vi "LaneExtractorHenesUseNetwork.vi"() -> ()   [LabVIEW 2024]
uses:
  <vilib>/userDefined/High Color/IMAQdx.ctl
  System.Windows.Forms
  <vilib>/Instr/_visa.llb/VISA Set IO Buffer Mask.ctl
  <vilib>/Instr/_visa.llb/VISA Flush IO Buffer Mask.ctl
  7dfa5429-d58f-460b-bb70-c7f4b3dcb04f.vi
  <vilib>/Instr/_visa.llb/VISA Configure Serial Port (Instr).vi
  <vilib>/Python/Open Venv Python Session.vi
  <vilib>/vision/driver/NI_Vision_Acquisition_Software.lvlib
panel:
  out "error out 2":errorcluster
  out "error out":errorcluster
  out "session out":refnum<k35>
  in  "ctelim":dbl=0.3 format="%#_13g"
  in  "GoBack":bool
  in  "Threshold":i32=1900
  in  "Spacing":i32=100
  in  "eps":i32=100
  in  "min_samples":i32=2
  in  "Ratio_Threshold":i32=4
  out "X_arrays":dbl[](array[numeric])=[-1100.0, -1100.0, -1120.0, -1120.0, -1140.0, -1140.0, -1140.0, -1160.0, -1160.0, -1160.0, -1180.0, -1180.0, -1180.0, -1200.0, -1200.0, -1200.0, -1220.0, -1220.0, -1220.0, -1220.0, -1240.0, -1260.0, -1260.0, -1260.0, -1280.0, -1280.0, -1280.0, -1300.0, -1300.0, -1300.0, -1320.0, -1320.0, -1320.0, -1340.0, -1340.0, -1340.0, -1360.0, -1360.0, -1360.0, -1380.0, -1380.0, -1380.0, -1400.0, -1400.0, -1400.0, -1420.0, -1420.0, -1440.0, -1440.0, -1460.0, -1460.0, -1460.0, -1480.0, -1480.0, -1480.0, -1480.0, -1500.0, -1500.0, -1500.0, -1520.0, -1520.0, -1520.0, -1540.0, -1540.0, -1540.0, -1560.0, -1560.0, -1560.0, -1580.0, -1580.0, -1600.0, -1600.0, -1620.0, -1620.0, -1620.0, -1640.0, -1640.0, -1640.0, -1660.0, -1660.0, -1680.0, -1680.0, -1680.0, -1700.0, -1700.0, -1700.0, -1720.0, -1720.0, -1740.0, -1740.0, -1760.0, -1760.0, -1780.0, -1780.0, -1780.0, -1800.0, -1820.0, -1820.0, -1820.0, -1840.0, -1840.0, -1860.0, -1860.0, -1880.0, -1880.0, -1900.0, -1900.0, -1920.0, -1940.0, -1960.0, -1960.0, -1980.0, -2000.0, -2000.0, -2040.0, -2060.0, -2060.0, -2080.0, -2120.0, -2120.0, -2140.0, -2140.0, -2160.0, -2180.0, -2200.0, -2220.0, -2220.0, -2260.0, -2280.0, -2300.0, -2320.0, -2340.0, -2360.0, -2380.0, -2400.0, -2420.0, -2460.0, -2500.0, -2520.0, -2540.0, -2580.0, -2980.0, -2980.0, -2960.0, -2940.0, -2960.0, 1180.0, 1200.0, 1220.0, 1220.0, 1240.0, 1260.0, 1260.0, 1280.0, 1380.0, 1380.0, 1380.0, 1400.0, 1400.0, 1420.0, 1420.0, 1440.0, 1460.0, 3460.0, 3460.0, 3460.0, 3460.0, 3460.0, 3480.0, 3480.0, 3500.0, -1657.163120567376, -2964.0, 1232.5, 1408.888888888889, 3470.0, 1252.0987654320988, 1271.6975308641975, 1291.2962962962963, 1310.8950617283951, 1330.4938271604938, 1350.0925925925926, 1369.6913580246915, 1389.29012345679]
  out "Y_arrays":dbl[](array[numeric])=[40.0, 60.0, 60.0, 80.0, 80.0, 100.0, 120.0, 120.0, 140.0, 160.0, 180.0, 200.0, 220.0, 220.0, 240.0, 260.0, 260.0, 280.0, 300.0, 320.0, 340.0, 360.0, 380.0, 400.0, 420.0, 440.0, 460.0, 460.0, 480.0, 500.0, 520.0, 540.0, 560.0, 560.0, 580.0, 600.0, 620.0, 640.0, 660.0, 660.0, 680.0, 700.0, 700.0, 720.0, 740.0, 760.0, 780.0, 800.0, 820.0, 840.0, 860.0, 880.0, 880.0, 900.0, 920.0, 940.0, 940.0, 960.0, 980.0, 980.0, 1000.0, 1020.0, 1020.0, 1040.0, 1060.0, 1080.0, 1100.0, 1120.0, 1140.0, 1160.0, 1180.0, 1200.0, 1220.0, 1240.0, 1260.0, 1260.0, 1280.0, 1300.0, 1320.0, 1340.0, 1360.0, 1380.0, 1400.0, 1420.0, 1440.0, 1460.0, 1480.0, 1500.0, 1520.0, 1540.0, 1560.0, 1580.0, 1600.0, 1620.0, 1640.0, 1660.0, 1700.0, 1720.0, 1740.0, 1760.0, 1780.0, 1800.0, 1820.0, 1860.0, 1880.0, 1900.0, 1940.0, 1960.0, 2000.0, 2040.0, 2080.0, 2120.0, 2140.0, 2160.0, 2240.0, 2260.0, 2300.0, 2340.0, 2400.0, 2420.0, 2460.0, 2480.0, 2520.0, 2560.0, 2600.0, 2660.0, 2700.0, 2740.0, 2800.0, 2840.0, 2880.0, 2940.0, 3000.0, 3060.0, 3100.0, 3160.0, 3240.0, 3300.0, 3360.0, 3420.0, 3500.0, 4340.0, 4360.0, 4380.0, 4380.0, 4460.0, 2560.0, 2580.0, 2560.0, 2540.0, 2540.0, 2540.0, 2520.0, 2520.0, 1720.0, 1700.0, 1680.0, 1680.0, 1660.0, 1660.0, 1640.0, 1660.0, 1660.0, 1800.0, 1780.0, 1760.0, 1740.0, 1720.0, 1720.0, 1700.0, 1700.0, 1330.354609929078, 4384.0, 2545.0, 1673.3333333333333, 1740.0, 2448.1481481481483, 2351.296296296296, 2254.4444444444443, 2157.5925925925926, 2060.740740740741, 1963.888888888889, 1867.037037037037, 1770.1851851851852]
  out "Clustered":T1={"appended array"=[-1100.0, -1100.0, -1120.0, -1120.0, -1140.0, -1140.0, -1140.0, -1160.0, -1160.0, -1160.0, -1180.0, -1180.0, -1180.0, -1200.0, -1200.0, -1200.0, -1220.0, -1220.0, -1220.0, -1220.0, -1240.0, -1260.0, -1260.0, -1260.0, -1280.0, -1280.0, -1280.0, -1300.0, -1300.0, -1300.0, -1320.0, -1320.0, -1320.0, -1340.0, -1340.0, -1340.0, -1360.0, -1360.0, -1360.0, -1380.0, -1380.0, -1380.0, -1400.0, -1400.0, -1400.0, -1420.0, -1420.0, -1440.0, -1440.0, -1460.0, -1460.0, -1460.0, -1480.0, -1480.0, -1480.0, -1480.0, -1500.0, -1500.0, -1500.0, -1520.0, -1520.0, -1520.0, -1540.0, -1540.0, -1540.0, -1560.0, -1560.0, -1560.0, -1580.0, -1580.0, -1600.0, -1600.0, -1620.0, -1620.0, -1620.0, -1640.0, -1640.0, -1640.0, -1660.0, -1660.0, -1680.0, -1680.0, -1680.0, -1700.0, -1700.0, -1700.0, -1720.0, -1720.0, -1740.0, -1740.0, -1760.0, -1760.0, -1780.0, -1780.0, -1780.0, -1800.0, -1820.0, -1820.0, -1820.0, -1840.0, -1840.0, -1860.0, -1860.0, -1880.0, -1880.0, -1900.0, -1900.0, -1920.0, -1940.0, -1960.0, -1960.0, -1980.0, -2000.0, -2000.0, -2040.0, -2060.0, -2060.0, -2080.0, -2120.0, -2120.0, -2140.0, -2140.0, -2160.0, -2180.0, -2200.0, -2220.0, -2220.0, -2260.0, -2280.0, -2300.0, -2320.0, -2340.0, -2360.0, -2380.0, -2400.0, -2420.0, -2460.0, -2500.0, -2520.0, -2540.0, -2580.0, -2980.0, -2980.0, -2960.0, -2940.0, -2960.0, 1180.0, 1200.0, 1220.0, 1220.0, 1240.0, 1260.0, 1260.0, 1280.0, 1380.0, 1380.0, 1380.0, 1400.0, 1400.0, 1420.0, 1420.0, 1440.0, 1460.0, 3460.0, 3460.0, 3460.0, 3460.0, 3460.0, 3480.0, 3480.0, 3500.0, -1657.163120567376, -2964.0, 1232.5, 1408.888888888889, 3470.0, 1252.0987654320988, 1271.6975308641975, 1291.2962962962963, 1310.8950617283951, 1330.4938271604938, 1350.0925925925926, 1369.6913580246915, 1389.29012345679], "appended array"=[40.0, 60.0, 60.0, 80.0, 80.0, 100.0, 120.0, 120.0, 140.0, 160.0, 180.0, 200.0, 220.0, 220.0, 240.0, 260.0, 260.0, 280.0, 300.0, 320.0, 340.0, 360.0, 380.0, 400.0, 420.0, 440.0, 460.0, 460.0, 480.0, 500.0, 520.0, 540.0, 560.0, 560.0, 580.0, 600.0, 620.0, 640.0, 660.0, 660.0, 680.0, 700.0, 700.0, 720.0, 740.0, 760.0, 780.0, 800.0, 820.0, 840.0, 860.0, 880.0, 880.0, 900.0, 920.0, 940.0, 940.0, 960.0, 980.0, 980.0, 1000.0, 1020.0, 1020.0, 1040.0, 1060.0, 1080.0, 1100.0, 1120.0, 1140.0, 1160.0, 1180.0, 1200.0, 1220.0, 1240.0, 1260.0, 1260.0, 1280.0, 1300.0, 1320.0, 1340.0, 1360.0, 1380.0, 1400.0, 1420.0, 1440.0, 1460.0, 1480.0, 1500.0, 1520.0, 1540.0, 1560.0, 1580.0, 1600.0, 1620.0, 1640.0, 1660.0, 1700.0, 1720.0, 1740.0, 1760.0, 1780.0, 1800.0, 1820.0, 1860.0, 1880.0, 1900.0, 1940.0, 1960.0, 2000.0, 2040.0, 2080.0, 2120.0, 2140.0, 2160.0, 2240.0, 2260.0, 2300.0, 2340.0, 2400.0, 2420.0, 2460.0, 2480.0, 2520.0, 2560.0, 2600.0, 2660.0, 2700.0, 2740.0, 2800.0, 2840.0, 2880.0, 2940.0, 3000.0, 3060.0, 3100.0, 3160.0, 3240.0, 3300.0, 3360.0, 3420.0, 3500.0, 4340.0, 4360.0, 4380.0, 4380.0, 4460.0, 2560.0, 2580.0, 2560.0, 2540.0, 2540.0, 2540.0, 2520.0, 2520.0, 1720.0, 1700.0, 1680.0, 1680.0, 1660.0, 1660.0, 1640.0, 1660.0, 1660.0, 1800.0, 1780.0, 1760.0, 1740.0, 1720.0, 1720.0, 1700.0, 1700.0, 1330.354609929078, 4384.0, 2545.0, 1673.3333333333333, 1740.0, 2448.1481481481483, 2351.296296296296, 2254.4444444444443, 2157.5925925925926, 2060.740740740741, 1963.888888888889, 1867.037037037037, 1770.1851851851852]}
  out "PythonLoop":u32=100
  in  "Looking X":i32=3500
  in  "Looking Y":i32=5200
  out "LookingAt":cluster{i32[], i32[]}={[700, 700, 3500, 3500, -3500, -3500, -700, -700, 700], [800, -800, -800, 5200, 5200, -800, -800, 800, 800]}
  out "Anthena_Steer":i32
  out "TargetDerection":cluster{dbl[], dbl[]}={[4.2861222383783204e-13, 0.0], [7000.0, 0.0]}
  out "VEstop":bool
  in  "length":dbl=1300.0
  out "PointCloud":T2(graph)=[{"appended array"=[700.0, 700.0, 3500.0, 3500.0, -3500.0, -3500.0, -700.0, -700.0, 700.0], "appended array"=[800.0, -800.0, -800.0, 5200.0, 5200.0, -800.0, -800.0, 800.0, 800.0]}, {"appended array"=[-560.0], "appended array"=[0.0]}, {"appended array"=[-450.0, -450.0, -800.0, -800.0, 0.0, 0.0, -450.0], "appended array"=[100.0, -300.0, -300.0, 1200.0, 1200.0, 100.0, 100.0]}, {"appended array"=[], "appended array"=[]}, {"appended array"=[450.0, 450.0, 800.0, 800.0, 0.0, 0.0, 450.0], "appended array"=[100.0, -300.0, -300.0, 1200.0, 1200.0, 100.0, 100.0]}, {"appended array"=[-1100.0, -1100.0, -1120.0, -1120.0, -1140.0, -1140.0, -1140.0, -1160.0, -1160.0, -1160.0, -1180.0, -1180.0, -1180.0, -1200.0, -1200.0, -1200.0, -1220.0, -1220.0, -1220.0, -1220.0, -1240.0, -1260.0, -1260.0, -1260.0, -1280.0, -1280.0, -1280.0, -1280.0, -1300.0, -1300.0, -1300.0, -1320.0, -1320.0, -1320.0, -1340.0, -1340.0, -1340.0, -1360.0, -1360.0, -1360.0, -1380.0, -1380.0, -1380.0, -1400.0, -1400.0, -1400.0, -1420.0, -1420.0, -1420.0, -1440.0, -1440.0, -1440.0, -1460.0, -1460.0, -1460.0, -1480.0, -1480.0, -1480.0, -1500.0, -1500.0, -1500.0, -1500.0, -1520.0, -1520.0, -1520.0, -1540.0, -1540.0, -1540.0, -1560.0, -1560.0, -1560.0, -1580.0, -1580.0, -1580.0, -1600.0, -1600.0, -1600.0, -1620.0, -1620.0, -1620.0, -1640.0, -1640.0, -1660.0, -1660.0, -1680.0, -1680.0, -1680.0, -1700.0, -1700.0, -1720.0, -1720.0, -1720.0, -1740.0, -1740.0, -1760.0, -1760.0, -1760.0, -1780.0, -1780.0, -1800.0, -1800.0, -1820.0, -1820.0, -1840.0, -1840.0, -1860.0, -1860.0, -1880.0, -1880.0, -1900.0, -1920.0, -1920.0, -1940.0, -1960.0, -1980.0, -2000.0, -2020.0, -2040.0, -2040.0, -2060.0, -2060.0, -2100.0, -2120.0, -2120.0, -2120.0, -2140.0, -2160.0, -2180.0, -2200.0, -2220.0, -2240.0, -2260.0, -2280.0, -2300.0, -2320.0, -2360.0, -2380.0, -2400.0, -2440.0, -2460.0, -2480.0, -2520.0, -2520.0, -2540.0, -2980.0, -2960.0, -2960.0, -2940.0, 1180.0, 1200.0, 1220.0, 1220.0, 1240.0, 1260.0, 1260.0, 1280.0, 1380.0, 1380.0, 1380.0, 1400.0, 1400.0, 1420.0, 1420.0, 1440.0, 1460.0, 3460.0, 3460.0, 3460.0, 3460.0, 3480.0, 3480.0, 3500.0, -1646.388888888889, -2960.0, 1232.5, 1408.888888888889, 3471.4285714285716, 1252.0987654320988, 1271.6975308641975, 1291.2962962962963, 1310.8950617283951, 1330.4938271604938, 1350.0925925925926, 1369.6913580246915, 1389.29012345679], "appended array"=[40.0, 60.0, 60.0, 80.0, 80.0, 100.0, 120.0, 120.0, 140.0, 160.0, 180.0, 200.0, 220.0, 220.0, 240.0, 260.0, 260.0, 280.0, 300.0, 320.0, 340.0, 360.0, 380.0, 400.0, 400.0, 420.0, 440.0, 460.0, 460.0, 480.0, 500.0, 520.0, 540.0, 560.0, 560.0, 580.0, 600.0, 620.0, 640.0, 660.0, 660.0, 680.0, 700.0, 700.0, 720.0, 740.0, 740.0, 760.0, 780.0, 780.0, 800.0, 820.0, 840.0, 860.0, 880.0, 880.0, 900.0, 920.0, 920.0, 940.0, 960.0, 980.0, 980.0, 1000.0, 1020.0, 1020.0, 1040.0, 1060.0, 1080.0, 1100.0, 1120.0, 1120.0, 1140.0, 1160.0, 1160.0, 1180.0, 1200.0, 1220.0, 1240.0, 1260.0, 1280.0, 1300.0, 1320.0, 1340.0, 1360.0, 1380.0, 1400.0, 1420.0, 1440.0, 1460.0, 1480.0, 1500.0, 1520.0, 1540.0, 1560.0, 1580.0, 1600.0, 1620.0, 1640.0, 1660.0, 1680.0, 1700.0, 1720.0, 1740.0, 1780.0, 1800.0, 1820.0, 1840.0, 1860.0, 1920.0, 1940.0, 1980.0, 2020.0, 2080.0, 2120.0, 2160.0, 2180.0, 2220.0, 2240.0, 2280.0, 2320.0, 2360.0, 2400.0, 2420.0, 2460.0, 2500.0, 2540.0, 2580.0, 2620.0, 2680.0, 2720.0, 2780.0, 2820.0, 2880.0, 2920.0, 2980.0, 3020.0, 3080.0, 3160.0, 3220.0, 3280.0, 3340.0, 3380.0, 3440.0, 4340.0, 4360.0, 4380.0, 4420.0, 2560.0, 2580.0, 2560.0, 2540.0, 2540.0, 2540.0, 2520.0, 2520.0, 1720.0, 1700.0, 1680.0, 1680.0, 1660.0, 1660.0, 1640.0, 1660.0, 1660.0, 1800.0, 1780.0, 1760.0, 1740.0, 1720.0, 1700.0, 1700.0, 1304.1666666666667, 4375.0, 2545.0, 1673.3333333333333, 1742.857142857143, 2448.1481481481483, 2351.296296296296, 2254.4444444444443, 2157.5925925925926, 2060.740740740741, 1963.888888888889, 1867.037037037037, 1770.1851851851852]}, {"appended array"=[4.2861222383783204e-13, 0.0], "appended array"=[7000.0, 0.0]}, {"appended array"=[450.0, 450.0, -450.0, -450.0, 450.0], "appended array"=[100.0, 950.0, 950.0, 100.0, 100.0]}]
  out "NearCarPointsLeft":cluster{"ROI_IN_X":dbl[], "ROI_IN_Y":dbl[]}={"ROI_IN_X"=[-560.0], "ROI_IN_Y"=[0.0]}
  out "NearCarROILeft":cluster{i32[], i32[]}={[-450, -450, -800, -800, 0, 0, -450], [100, -300, -300, 1200, 1200, 100, 100]}
  out "NearCarPointsRight":cluster{"ROI_IN_X":dbl[], "ROI_IN_Y":dbl[]}
  out "NearCarROIRight":cluster{i32[], i32[]}={[450, 450, 800, 800, 0, 0, 450], [100, -300, -300, 1200, 1200, 100, 100]}
  out "NearSteer":dbl=71.42857142857143
  out "TooClose":bool=TRUE
  out "GobackROI":cluster{i32[], i32[]}={[450, 450, -450, -450, 450], [100, 950, 950, 100, 100]}
  in  "LiDAR":refnum<visa-resource-name>="COM3"
  out "Clustering Error":errorcluster
  out "read buffer":string
  out "LidarLoop":u32=100
  in  "격자크기":dbl=20.0
  out "X_arraysREAL":i32[](array[numeric])=[260, 240, 200, 220, 220, 240, 100, 80, 60]
  out "Y_arraysREAL":i32[](array[numeric])=[-120, -120, -120, -120, -140, -140, -80, -60, -60]
  in  "Current_image":refnum<k24>(container)
  in  "Right_lane":refnum<k24>(container)
  in  "Left_lane":refnum<k24>(container)
  out "inference time":string="Total: 586.3ms"
  out "error out 3":errorcluster
  out "Image_String":string
  in  "File Path":path=path "C:/Users/JungiHong/OneDrive/Hongik/HI-RACE/2026-01/platform_1_5/ExperimentModules/LaneTracking/forTrainImages/frame_014.jpg"
  in  "UseVideo":bool=TRUE
  in  "Cam No.":T3="cam3"
  in  "input_spd":i16
  in  "HENES":refnum<visa-resource-name>="COM4"
  out "E-STOP":bool
  out "Remote_M/A":bool
  out "Steer_Feed":dbl
  out "Alive_PCU":u8(slide) scale=0.0..254.0
  out "Gear_Feed":u8
  out "Speed_Feed(RPM)":dbl format="%#_g rpm"
  out "버퍼 읽기":string
  out "Speed_Feed(m/s)":dbl
  in  "HLV_Gear":u8
  in  "HLV_A/M":bool=TRUE
  in  "HLV_E-stop":bool
  out "HENES Loop Time":u32=19
  in  "v(Velocity)m/s":dbl=1.0
  in  "k(Gain)":dbl=1.0
  out "δ(OutputSteer)degrees":dbl=3.1742774367668782
  out "changearray":u32=2
  out "CV Loop Time":u32=19558436
  in  "stop":bool
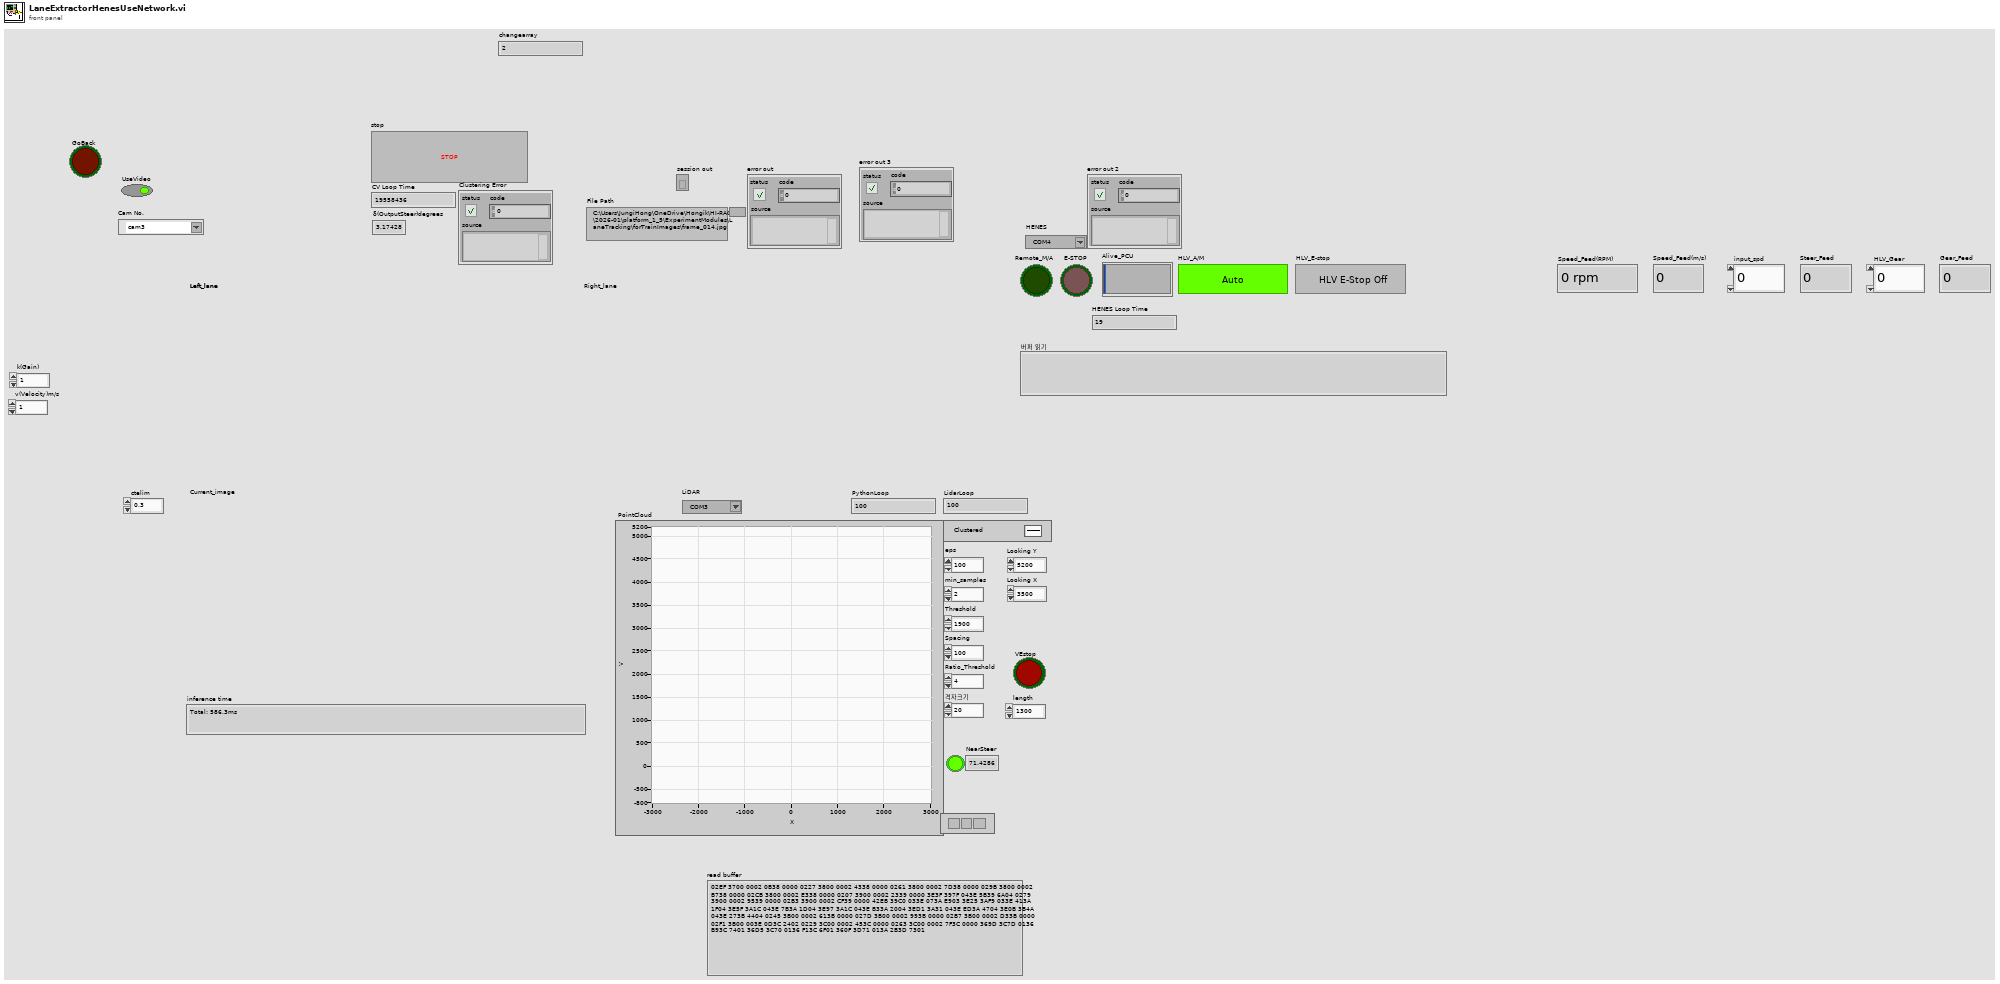
[diagram p1: front panel]
types:
  T1 = cluster{"appended array":dbl[], "appended array":dbl[]}
  T2 = cluster{"appended array":dbl[], "appended array":dbl[]}[]
  T3 = typedef "IMAQdx.ctl" = refnum<k21>
  T4 = cluster{"HENES_M/A":u8, "HENES_E-Stop":u8, "HENES_Gear":u8, "HENES_Speed":i16, "HENES_Steer":i16, "HENES_Alive":u8}
  T5 = typedef "VISA Flush IO Buffer Mask.ctl" = u16
  T6 = typedef "VISA Set IO Buffer Mask.ctl" = u16
  T7 = cluster{"HLV_M/A_Status":u8, "HLV_E-Stop":u8, "HLV_Gear":u8, "HLV_Speed":i16, "HLV_Steer":i16, "HLV_Alive":u8}
  T8 = typedef "IMAQ Image.ctl" = refnum<image>
  T9 = cluster{"Global Rectangle":i32[], "Contours":cluster{"ID":enum32{"External", "Internal"}, "Type":u32, "Coordinates":i32[]}[]}
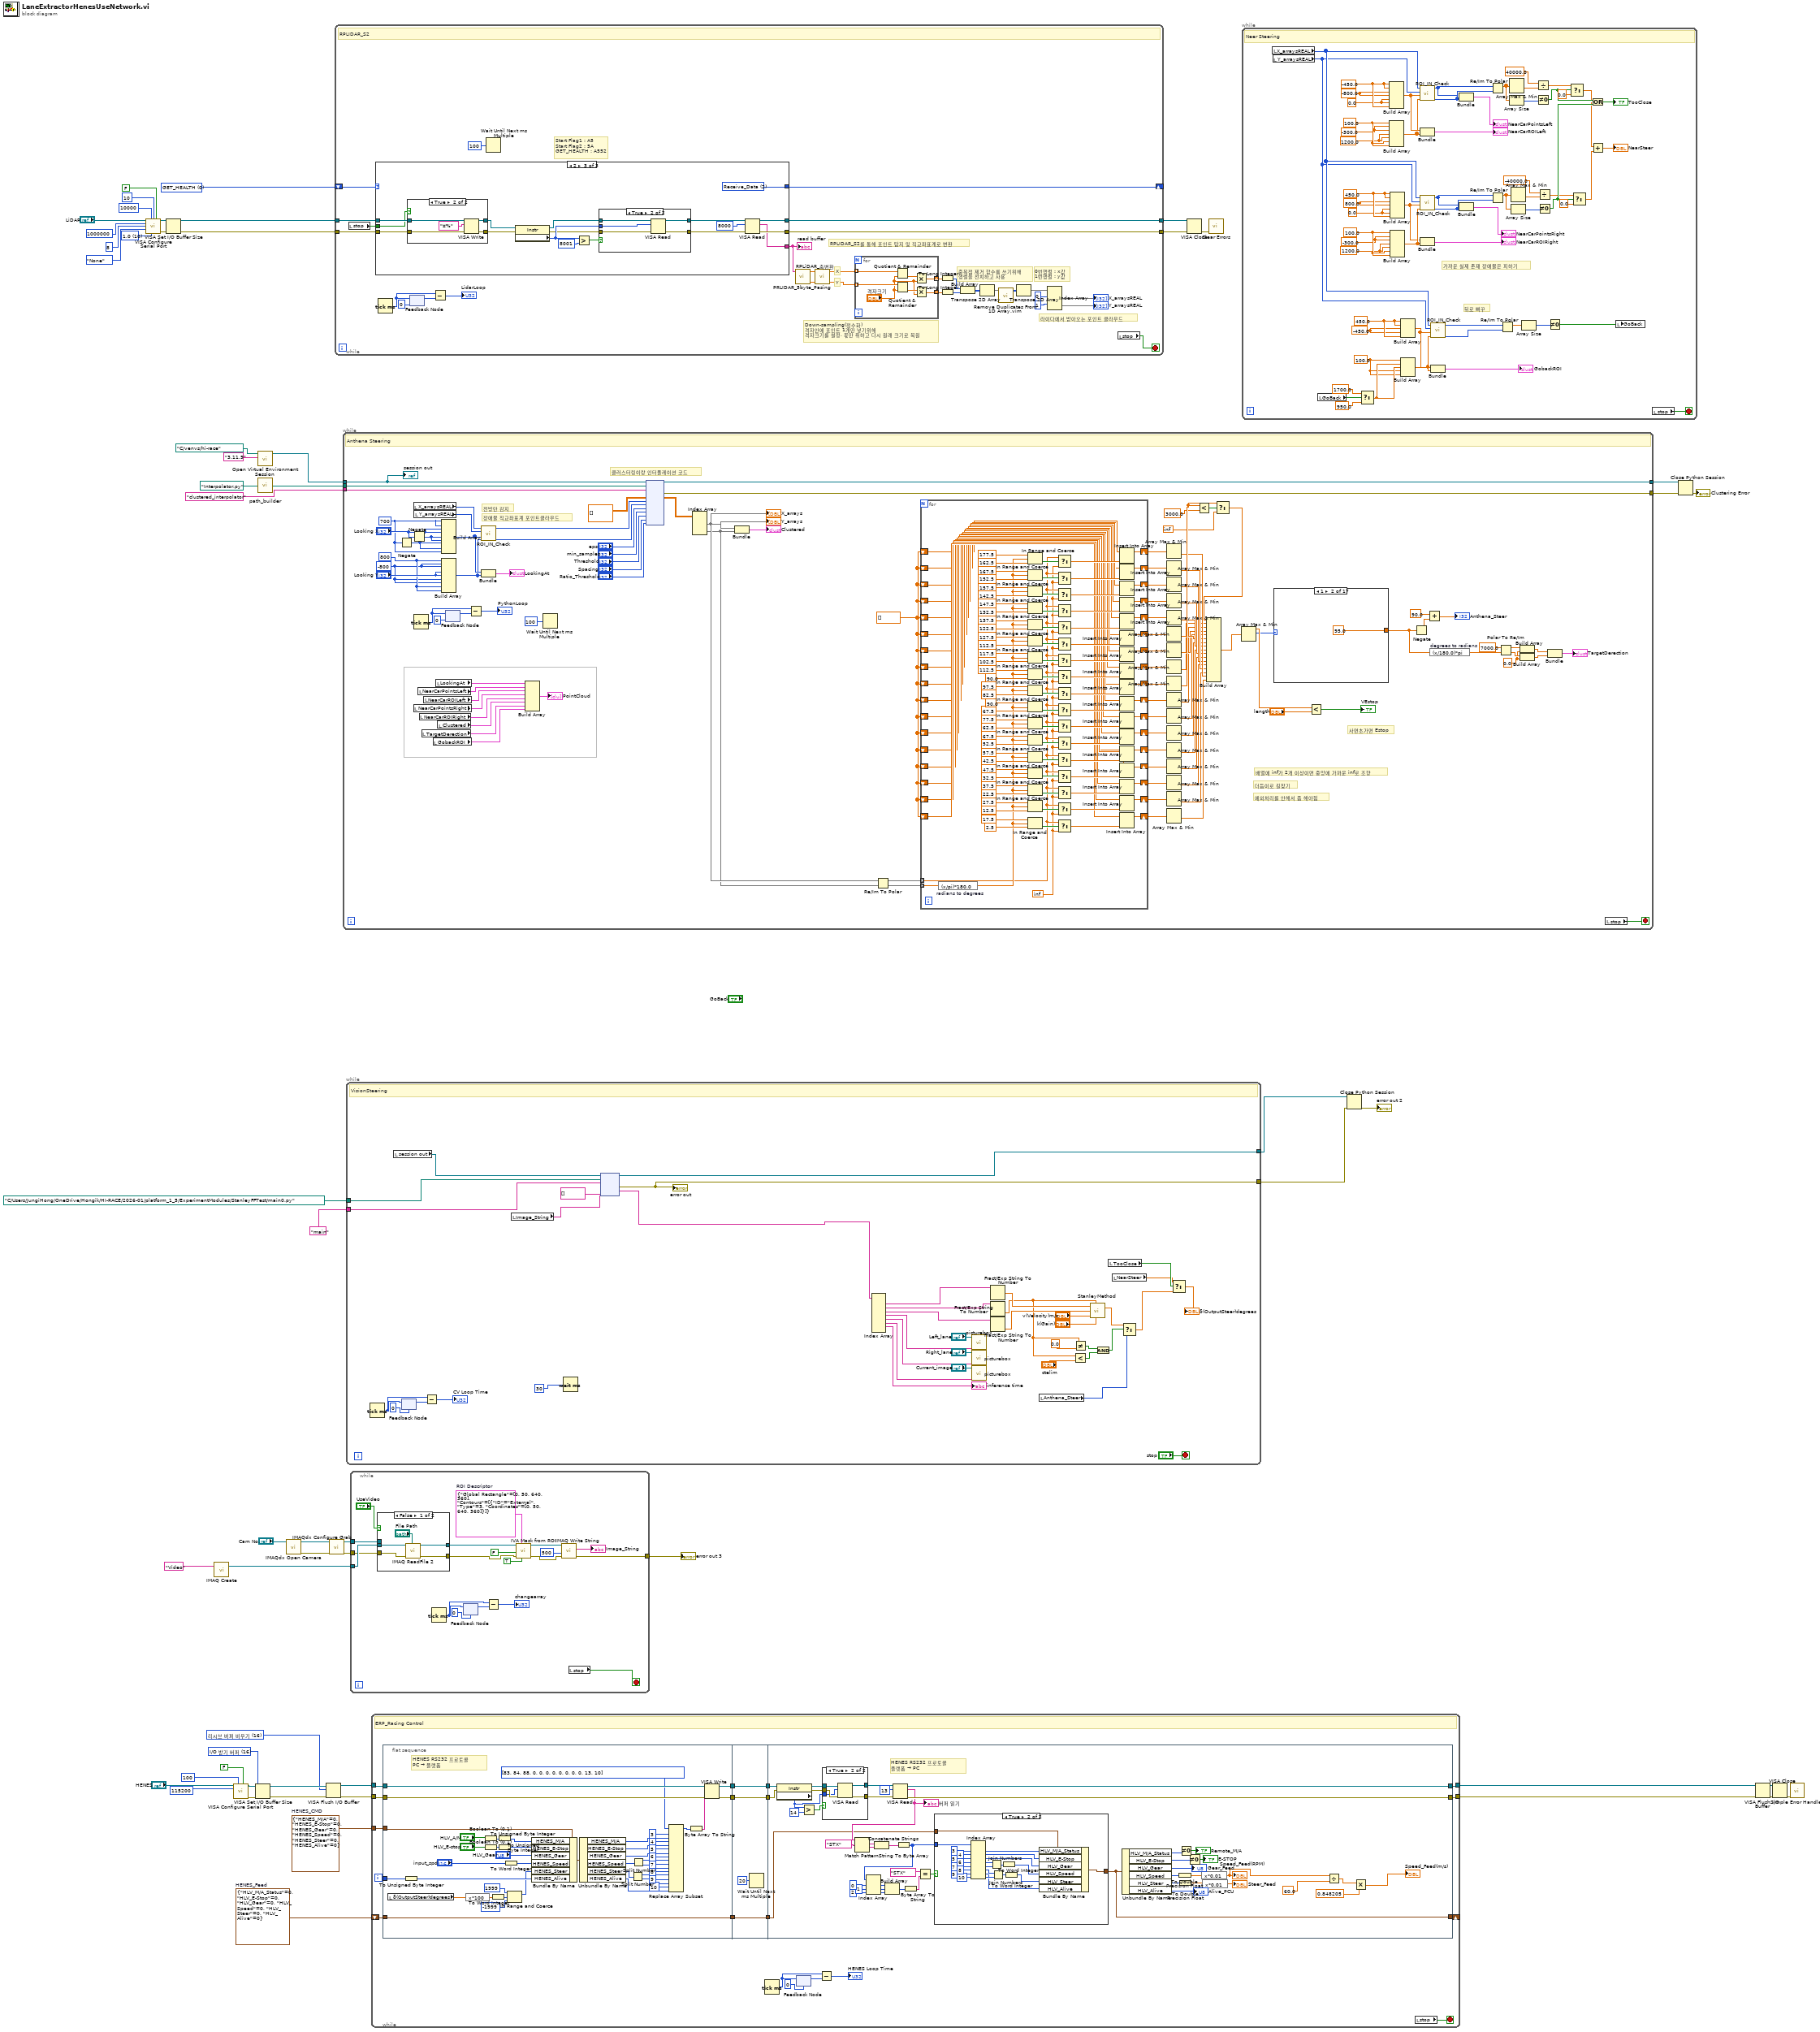
[diagram p0: block diagram]
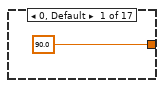
[diagram p2: hidden frame]
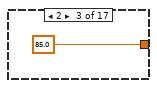
[diagram p3: hidden frame]
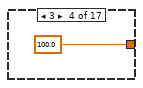
[diagram p4: hidden frame]
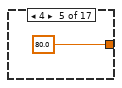
[diagram p5: hidden frame]
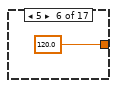
[diagram p6: hidden frame]
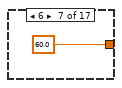
[diagram p7: hidden frame]
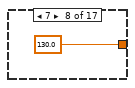
[diagram p8: hidden frame]
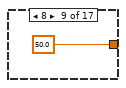
[diagram p9: hidden frame]
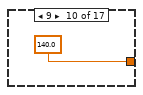
[diagram p10: hidden frame]
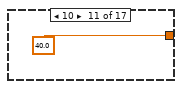
[diagram p11: hidden frame]
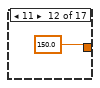
[diagram p12: hidden frame]
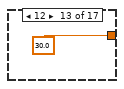
[diagram p13: hidden frame]
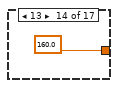
[diagram p14: hidden frame]
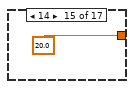
[diagram p15: hidden frame]
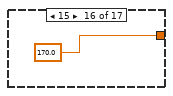
[diagram p16: hidden frame]
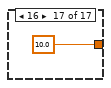
[diagram p17: hidden frame]
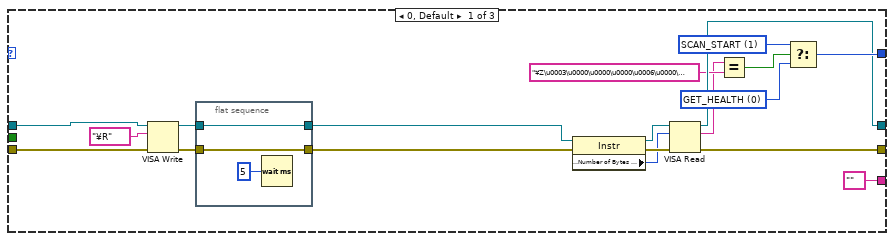
[diagram p18: hidden frame]
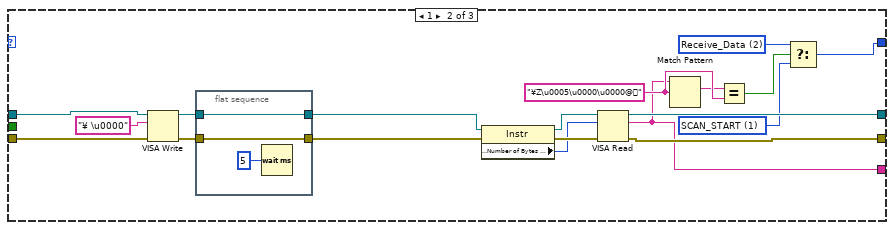
[diagram p19: hidden frame]
diagram:
  w16 = u16 10 items=["1.0"=10, "1.5"=15, "2.0"=20] ("stop bits (10: 1 bit)")
  w18 = u16 0 items=["GET_HEALTH", "SCAN_START", "Receive_Data"]
  w38 = T4 {"HENES_M/A"=0, "HENES_E-Stop"=0, "HENES_Gear"=0, "HENES_Speed"=0, "HENES_Steer"=0, "HENES_Alive"=0}  # HENES_CMD
  w41 = T5 16 items=["리시브 버퍼 비우기"=16, "전달 버퍼 디바이스에 쓰기"=32, "리시브 버퍼 비우기(I/O 없음)"=64, "전달 버퍼 비우기"=128] ("Mask")
  w44 = T6 16 items=["I/O 받기 버퍼"=16, "I/O 전달 버퍼"=32, "I/O 받기와 전달 버퍼"=48] ("Mask")
  w48 = T7 {"HLV_M/A_Status"=0, "HLV_E-Stop"=0, "HLV_Gear"=0, "HLV_Speed"=0, "HLV_Steer"=0, "HLV_Alive"=0}  # HENES_Feed
  n1 = call-poly "VISA Configure Serial Port"("VISA resource name"="LiDAR", "timeout (10sec)"=u32 10000, "termination char\n(0xA = '\\n' = LF)"=u8 10 ("termination char\n(0xA = '\\n' = LF)"), "Enable Termination\nChar (T)"=FALSE ("Enable Termination\nChar (T)"), "baud rate (9600)"=u32 1000000, "data bits (8)"=u16 8, "parity (0:none)"=enum16{"None", "Odd", "Even", "Mark", "Space"}."None", "stop bits (10: 1 bit)"=w16) -> ("VISA resource name out"=w25:refnum<visa-resource-name>, "error out"=w24:errorcluster)  [unwired: 6 in]
  n2 = VISA Set I/O Buffer Size(VISA resource name=w25, error in (no error)=w24) -> (VISA resource name out=w20:refnum<visa-resource-name>, error out=w19:errorcluster)  [unwired: 2 in]
  n3 = call "IMAQ Create"("Image Name"="Video") -> ("New Image"=w56:T8)  [unwired: 4 in, 1 out]
  n4 = call-poly "VISA Configure Serial Port"("VISA resource name"="HENES", "timeout (10sec)"=u32 100, "Enable Termination\nChar (T)"=FALSE ("Enable Termination\nChar (T)"), "baud rate (9600)"=u32 115200) -> ("VISA resource name out"=w40:refnum<visa-resource-name>, "error out"=w39:errorcluster)  [unwired: 10 in]
  n5 = VISA Set I/O Buffer Size(VISA resource name=w40, mask (16)=w44, error in (no error)=w39) -> (VISA resource name out=w43:refnum<visa-resource-name>, error out=w42:errorcluster)  [unwired: 1 in]
  n6 = call-poly <vilib>:"Open Virtual Environment Session.vi"("Python version"="3.11.9", "Env path"=path "C:/venvs/hi-race" ("Name")) -> ("session out"=w7:refnum<k35>)  [unwired: 8 in, 1 out]
  n7 = call "path_builder.vi"("Name"=path "Interpolator.py") -> ("appended path"=w11:path)
  n8 = call <vilib>:"IMAQdx Open Camera.vi"("Session In"="Cam No.") -> ("error out"=w34:errorcluster, "Session Out"=w35:T3)  [unwired: 9 in]
  n9 = VISA Flush I/O Buffer(VISA resource name=w43, mask (16)=w41, error in (no error)=w42) -> (VISA resource name out=w53:refnum<visa-resource-name>, error out=w52:errorcluster)
  n10 = call <vilib>:"IMAQdx Configure Grab.vi"("error in"=w34, "Session In"=w35) -> ("error out"=w33:errorcluster, "Session Out"=w36:T3)  [unwired: 8 in]
  n11 = while {
    tunnel: [w77] -> w29
    tunnel: [w78] -> w28
    tunnel: w20 -> [w86]
    tunnel: w19 -> [w85]
    shift-right: [w84] -> _
    shift-left: w18 -> [w87]
    stop <- w58 stop-if-true
    # "라이다에서 받아오는 포인트 클라우드"
    # "RPLIDAR_S2를 통해 포인트 탐지 및 직교좌표계로 변환"
    # "Start Flag1 : A5\nStart Flag2 : 5A \nGET_HEALTH : A552"
    # "0번행렬 : x값\n1번행렬 : y값"
    # "중복점 제거 함수를 쓰기위해\n행렬을 전치하고 사용"
    # "Down-sampling(정수화)\n격자안에 포인트 1개만 넣기위해\n격자크기를 설정, 몫만 취하고 다시 원래 크기로 복원"
    # "Y"
    # "X"
    # "RPLIDAR_S2"
    n12 = local read "stop"() -> (w83:bool)
    n13 = case shown="2" w87 {
      tunnel: w86 -> [w112 w130 w153]
      tunnel: w85 -> [w111 w129 w152]
      tunnel: [w113 w126 w139] -> w84
      tunnel: [w102 w127 w155] -> w78
      tunnel: [w101 w128 w154] -> w77
      tunnel: w83 -> [_ _ w151]
      tunnel: ["" ("read buffer") w124 w150] -> w62
      frame 0, Default {
        w95 = u16 0 items=["GET_HEALTH", "SCAN_START", "Receive_Data"]
        w96 = u16 1 items=["GET_HEALTH", "SCAN_START", "Receive_Data"]
        n14 = VISA Write(VISA resource name=w112, write buffer="¥R", error in (no error)=w111) -> (VISA resource name out=w106:refnum<visa-resource-name>, error out=w105:errorcluster)  [unwired: 1 out]
        n15 = flat-sequence {
          tunnel: w106 -> [w115]
          tunnel: w105 -> [w114]
          tunnel: [w115] -> w104
          tunnel: [w114] -> w103
          frame #0 {
            n16 = Wait (ms)(milliseconds to wait=u32 5 ("대기 시간 (ms)")) -> ()  [unwired: 1 out]
          }
        }
        n17 = property class="Instr"(reference=w104, error in=w103) -> (reference out=w109:refnum<visa-resource-name>, error out=w108:errorcluster, "Serial Settings:Number of Bytes at Serial Port"=w107:u32)
        n18 = VISA Read(VISA resource name=w109, byte count=w107, error in (no error)=w108) -> (VISA resource name out=w101:refnum<visa-resource-name>, read buffer=w98:string, error out=w102:errorcluster)  [unwired: 1 out]
        n19 = Equal?(x=w98, y="¥Z\u0003\u0000\u0000\u0000\u0006\u0000\u0000\u0000") -> (x = y?=w99:bool)
        n20 = Select(t=w96, s=w99, f=w95) -> (s? t:f=w113:u16)
      }
      frame 1 {
        w117 = u16 2 items=["GET_HEALTH", "SCAN_START", "Receive_Data"]
        w118 = u16 1 items=["GET_HEALTH", "SCAN_START", "Receive_Data"]
        w131 = "¥Z\u0005\u0000\u0000@"
        n21 = VISA Write(VISA resource name=w130, write buffer="¥ \u0000", error in (no error)=w129) -> (VISA resource name out=w133:refnum<visa-resource-name>, error out=w134:errorcluster)  [unwired: 1 out]
        n22 = flat-sequence {
          tunnel: w133 -> [w137]
          tunnel: w134 -> [w136]
          tunnel: [w137] -> w120
          tunnel: [w136] -> w119
          frame #0 {
            n23 = Wait (ms)(milliseconds to wait=u32 5 ("대기 시간 (ms)")) -> ()  [unwired: 1 out]
          }
        }
        n24 = property class="Instr"(reference=w120, error in=w119) -> (reference out=w123:refnum<visa-resource-name>, error out=w122:errorcluster, "Serial Settings:Number of Bytes at Serial Port"=w121:u32)
        n25 = VISA Read(VISA resource name=w123, byte count=w121, error in (no error)=w122) -> (VISA resource name out=w128:refnum<visa-resource-name>, read buffer=w124:string, error out=w127:errorcluster)  [unwired: 1 out]
        n26 = Match Pattern(string=w124, regular expression=w131) -> (match substring=w125:string)  [unwired: 1 in, 3 out]
        n27 = Equal?(x=w125, y=w131) -> (x = y?=w135:bool)
        n28 = Select(t=w117, s=w135, f=w118) -> (s? t:f=w126:u16)
      }
      frame 2 {
        w139 = u16 2 items=["GET_HEALTH", "SCAN_START", "Receive_Data"]
        n29 = case shown="True" w151 {
          tunnel: w153 -> [w164 w168]
          tunnel: w152 -> [w163 w167]
          tunnel: [w164 w166] -> w149
          tunnel: [w163 w165] -> w148
          frame False {
          }
          frame True {
            n30 = VISA Write(VISA resource name=w168, write buffer="¥%", error in (no error)=w167) -> (VISA resource name out=w166:refnum<visa-resource-name>, error out=w165:errorcluster)  [unwired: 1 out]
          }
        }
        n31 = property class="Instr"(reference=w149, error in=w148) -> (reference out=w144:refnum<visa-resource-name>, error out=w143:errorcluster, "Serial Settings:Number of Bytes at Serial Port"=w145:u32)
        n32 = Greater?(x=w145, y=u32 8001) -> (0:w147:bool)
        n33 = case shown="True" w147 {
          tunnel: w144 -> [w157 w162]
          tunnel: w145 -> [_ w161]
          tunnel: w143 -> [w156 w160]
          tunnel: [w157 w159] -> w142
          tunnel: [w156 w158] -> w141
          frame False {
          }
          frame True {
            n34 = VISA Read(VISA resource name=w162, byte count=w161, error in (no error)=w160) -> (VISA resource name out=w159:refnum<visa-resource-name>, error out=w158:errorcluster)  [unwired: 2 out]
          }
        }
        n35 = VISA Read(VISA resource name=w142, byte count=u32 8000, error in (no error)=w141) -> (VISA resource name out=w154:refnum<visa-resource-name>, read buffer=w150:string, error out=w155:errorcluster)  [unwired: 1 out]
      }
    }
    "read buffer" <- w62
    n36 = Tick Count (ms)() -> (millisecond timer value=w82:u32)
    n37 = feedback #1(u32 0 ("millisecond timer value")) -> (w81:u32)
    n38 = feedback-in #1(w82) -> ()
    n39 = Subtract(x=w82, y=w81) -> (x-y=→"LidarLoop":u32)
    n40 = Wait Until Next ms Multiple(millisecond multiple=u32 100) -> ()  [unwired: 1 out]
    n41 = call "PRLIDAR_5byte_Pasing.vi"("RPLIDAR_Data"=w62) -> ("Theta(deg)"=w65:dbl[], "Distance(mm)"=w66:dbl[])  [unwired: 9 in]
    n42 = call "RPLiDAR_축변환.vi"("Theta(deg)"=w65, "Distance(mm)"=w66) -> ("Y"=w63:dbl[], "X"=w64:dbl[])  [unwired: 8 in]
    n43 = for {
      tunnel: w64 -> [w94] mode=indexing
      tunnel: w63 -> [w93] mode=indexing
      tunnel: [w90] -> w75 mode=indexing
      tunnel: [w89] -> w76 mode=indexing
      n44 = Quotient & Remainder(x=w94, y="격자크기") -> (floor(x/y)=w92:dbl)  [unwired: 1 out]
      n45 = Quotient & Remainder(x=w93, y="격자크기") -> (floor(x/y)=w91:dbl)  [unwired: 1 out]
      n46 = Multiply(x=w92, y="격자크기") -> (x*y=w90:dbl)
      n47 = Multiply(x=w91, y="격자크기") -> (x*y=w89:dbl)
    }
    n48 = To Long Integer(number=w75) -> (32bit integer=w70:i32[])
    n49 = To Long Integer(number=w76) -> (32bit integer=w69:i32[])
    n50 = Build Array(w70, w69) -> (w71:i32[][])
    n51 = Transpose 2D Array(2D array=w71) -> (transposed array=w67:i32[][])
    n52 = call "Remove Duplicates From 1D Array.vim"("array"=w67) -> ("array with duplicates removed"=w68:i32[][])  [unwired: 10 in]
    n53 = Transpose 2D Array(2D array=w68) -> (transposed array=w72:i32[][])
    n54 = Index Array(array=w72, index (row) #1=0 ("index (row)"), index (row) #2=1 ("index (row)")) -> (element #1=→"X_arraysREAL":i32[], element #2=→"Y_arraysREAL":i32[])  [unwired: 2 in]
    n55 = local read "stop"() -> (w58:bool)
  }
  n56 = while {
    tunnel: [w271] -> w15
    tunnel: "clustered_interpolator" ("function name") -> [w269]
    tunnel: w11 -> [w268]
    tunnel: w7 -> [w170]
    tunnel: [w270] -> w14
    stop <- w180 stop-if-true
    w183 = dbl[] []
    w185 = 0.0 ("r")
    w245 = -800
    w246 = 800
    w247 = 700
    # "사면초가면 Estop"
    # "배열에 inf가 2개 이상이면 중앙에 가까운 inf로 조향"
    # "예외처리를 안해서 좀 해야됨"
    # "더듬이로 길찾기"
    # "전방만 감지"
    # "장애물 직교좌표계 포인트클라우드"
    # "클러스터링이랑 인터폴레이션 코드"
    # "Anthena Steering"
    n57 = Negate(x=w247) -> (-x=w250:i32)
    n58 = Negate(x="Looking X") -> (-x=w251:i32)
    n59 = local read "X_arraysREAL"() -> (w244:i32[])
    n60 = local read "NearCarPointsRight"() -> (w177:cluster{"ROI_IN_X":dbl[], "ROI_IN_Y":dbl[]})
    n61 = local read "Y_arraysREAL"() -> (w243:i32[])
    n62 = Tick Count (ms)() -> (millisecond timer value=w255:u32)
    n63 = local read "NearCarPointsLeft"() -> (w174:cluster{"ROI_IN_X":dbl[], "ROI_IN_Y":dbl[]})
    n64 = local read "NearCarROIRight"() -> (w178:cluster{i32[], i32[]})
    n65 = local read "TargetDerection"() -> (w172:cluster{dbl[], dbl[]})
    n66 = local read "NearCarROILeft"() -> (w175:cluster{i32[], i32[]})
    n67 = local read "GobackROI"() -> (w171:cluster{i32[], i32[]})
    n68 = local read "LookingAt"() -> (w173:cluster{i32[], i32[]})
    n69 = local read "Clustered"() -> (w179:T1)
    n70 = Build Array(w247, w247, "Looking X", "Looking X", w251, w251, w250, w250, w247) -> (w253:i32[])
    n71 = Build Array(w246, w245, w245, "Looking Y", "Looking Y", w245, w245, w246, w246) -> (w252:i32[])
    n72 = feedback #2(u32 0 ("millisecond timer value")) -> (w256:u32)
    n73 = feedback-in #2(w255) -> ()
    n74 = Subtract(x=w255, y=w256) -> (x-y=→"PythonLoop":u32)
    n75 = call "ROI_IN_Check.vi"("도형Y좌표"=w252, "도형X좌표"=w253, "LiDAR_Y"=w243, "LiDAR_X"=w244) -> ("ROI_IN_Y"=w241:i32[], "ROI_IN_X"=w242:i32[])  [unwired: 6 in]
    n76 = Bundle(w253, w252) -> (→"LookingAt":cluster{i32[], i32[]})  [unwired: 1 in]
    n77 = Build Array(w173, w174, w175, w177, w178, w179, w172, w171) -> (→"PointCloud":T2)
    n78 = Wait Until Next ms Multiple(millisecond multiple=u32 100) -> ()  [unwired: 1 out]
    n79 = node(w170, w268, w269, dbl[][] [] ("appended array"), w242, w241, "eps", "min_samples", "Threshold", "Spacing", "Ratio_Threshold") -> (w270:refnum<k35>, w271:errorcluster, w267:dbl[][])  [unwired: 8 in, 2 out]
    n80 = Index Array(array=w267) -> (element #1=w182:dbl[], element #2=w181:dbl[])  [unwired: 4 in]
    "X_arrays" <- w182
    "Y_arrays" <- w181
    n81 = Bundle("appended array"=w182, "appended array"=w181) -> (→"Clustered":T1)  [unwired: 1 in]
    n82 = Re/Im To Polar(2:w181, 3:w182) -> (0:w189:dbl[], 1:w190:dbl[])
    n83 = for {
      tunnel: w189 -> [w394] mode=indexing
      tunnel: w190 -> [w316] mode=indexing
      shift-right: [w361] -> w191
      shift-left: w183 -> [w293]
      shift-right: [w360] -> w192
      shift-left: w183 -> [w294]
      shift-right: [w359] -> w193
      shift-left: w183 -> [w295]
      shift-right: [w358] -> w194
      shift-left: w183 -> [w296]
      shift-right: [w357] -> w195
      shift-left: w183 -> [w297]
      shift-right: [w356] -> w196
      shift-left: w183 -> [w298]
      shift-right: [w355] -> w197
      shift-left: w183 -> [w299]
      shift-right: [w354] -> w198
      shift-left: w183 -> [w300]
      shift-right: [w350] -> w204
      shift-left: w183 -> [w301]
      shift-right: [w314] -> w219
      shift-left: w183 -> [w302]
      shift-right: [w313] -> w220
      shift-left: w183 -> [w303]
      shift-right: [w312] -> w221
      shift-left: w183 -> [w304]
      shift-right: [w311] -> w222
      shift-left: w183 -> [w305]
      shift-right: [w307] -> w226
      shift-left: w183 -> [w289]
      shift-right: [w308] -> w225
      shift-left: w183 -> [w290]
      shift-right: [w309] -> w224
      shift-left: w183 -> [w291]
      shift-right: [w310] -> w223
      shift-left: w183 -> [w292]
      w315 = inf
      n84 = expression code="(x/pi)*180.0" "radians to degrees"(w394) -> (w334:dbl)
      n85 = In Range and Coerce(upper limit=177.5, x=w334, lower limit=162.5) -> (In Range?=w321:bool)  [unwired: 1 out]
      n86 = In Range and Coerce(upper limit=167.5, x=w334, lower limit=152.5 ("upper limit")) -> (In Range?=w322:bool)  [unwired: 1 out]
      n87 = In Range and Coerce(upper limit=157.5 ("lower limit"), x=w334, lower limit=142.5 ("upper limit")) -> (In Range?=w323:bool)  [unwired: 1 out]
      n88 = In Range and Coerce(upper limit=147.5 ("lower limit"), x=w334, lower limit=132.5 ("upper limit")) -> (In Range?=w324:bool)  [unwired: 1 out]
      n89 = In Range and Coerce(upper limit=137.5, x=w334, lower limit=122.5) -> (In Range?=w375:bool)  [unwired: 1 out]
      n90 = In Range and Coerce(upper limit=127.5, x=w334, lower limit=112.5) -> (In Range?=w377:bool)  [unwired: 1 out]
      n91 = In Range and Coerce(upper limit=117.5, x=w334, lower limit=102.5) -> (In Range?=w373:bool)  [unwired: 1 out]
      n92 = In Range and Coerce(upper limit=112.5, x=w334, lower limit=90.0) -> (In Range?=w372:bool)  [unwired: 1 out]
      n93 = In Range and Coerce(upper limit=97.5, x=w334, lower limit=82.5) -> (In Range?=w371:bool)  [unwired: 1 out]
      n94 = In Range and Coerce(upper limit=90.0, x=w334, lower limit=67.5) -> (In Range?=w370:bool)  [unwired: 1 out]
      n95 = In Range and Coerce(upper limit=77.5, x=w334, lower limit=62.5) -> (In Range?=w369:bool)  [unwired: 1 out]
      n96 = In Range and Coerce(upper limit=67.5, x=w334, lower limit=52.5) -> (In Range?=w368:bool)  [unwired: 1 out]
      n97 = In Range and Coerce(upper limit=57.5, x=w334, lower limit=42.5) -> (In Range?=w353:bool)  [unwired: 1 out]
      n98 = In Range and Coerce(upper limit=47.5, x=w334, lower limit=32.5) -> (In Range?=w332:bool)  [unwired: 1 out]
      n99 = In Range and Coerce(upper limit=37.5, x=w334, lower limit=22.5) -> (In Range?=w331:bool)  [unwired: 1 out]
      n100 = In Range and Coerce(upper limit=27.5, x=w334, lower limit=12.5) -> (In Range?=w330:bool)  [unwired: 1 out]
      n101 = In Range and Coerce(upper limit=17.5, x=w334, lower limit=2.5) -> (In Range?=w329:bool)  [unwired: 1 out]
      n102 = Select(t=w316, s=w321, f=w315) -> (s? t:f=w320:dbl)
      n103 = Select(t=w316, s=w322, f=w315) -> (s? t:f=w319:dbl)
      n104 = Select(t=w316, s=w323, f=w315) -> (s? t:f=w318:dbl)
      n105 = Select(t=w316, s=w324, f=w315) -> (s? t:f=w317:dbl)
      n106 = Select(t=w316, s=w375, f=w315) -> (s? t:f=w374:dbl)
      n107 = Select(t=w316, s=w377, f=w315) -> (s? t:f=w376:dbl)
      n108 = Select(t=w316, s=w373, f=w315) -> (s? t:f=w362:dbl)
      n109 = Select(t=w316, s=w372, f=w315) -> (s? t:f=w363:dbl)
      n110 = Select(t=w316, s=w371, f=w315) -> (s? t:f=w364:dbl)
      n111 = Select(t=w316, s=w370, f=w315) -> (s? t:f=w365:dbl)
      n112 = Select(t=w316, s=w369, f=w315) -> (s? t:f=w366:dbl)
      n113 = Select(t=w316, s=w368, f=w315) -> (s? t:f=w367:dbl)
      n114 = Select(t=w316, s=w353, f=w315) -> (s? t:f=w333:dbl)
      n115 = Select(t=w316, s=w332, f=w315) -> (s? t:f=w328:dbl)
      n116 = Select(t=w316, s=w331, f=w315) -> (s? t:f=w327:dbl)
      n117 = Select(t=w316, s=w330, f=w315) -> (s? t:f=w326:dbl)
      n118 = Select(t=w316, s=w329, f=w315) -> (s? t:f=w325:dbl)
      n119 = Insert Into Array(array=w289, new element=w320) -> (w307:dbl[])  [unwired: 1 in]
      n120 = Insert Into Array(array=w290, new element=w319) -> (w308:dbl[])  [unwired: 1 in]
      n121 = Insert Into Array(array=w291, new element=w318) -> (w309:dbl[])  [unwired: 1 in]
      n122 = Insert Into Array(array=w292, new element=w317) -> (w310:dbl[])  [unwired: 1 in]
      n123 = Insert Into Array(array=w293, new element=w374) -> (w361:dbl[])  [unwired: 1 in]
      n124 = Insert Into Array(array=w294, new element=w376) -> (w360:dbl[])  [unwired: 1 in]
      n125 = Insert Into Array(array=w295, new element=w362) -> (w359:dbl[])  [unwired: 1 in]
      n126 = Insert Into Array(array=w296, new element=w363) -> (w358:dbl[])  [unwired: 1 in]
      n127 = Insert Into Array(array=w297, new element=w364) -> (w357:dbl[])  [unwired: 1 in]
      n128 = Insert Into Array(array=w298, new element=w365) -> (w356:dbl[])  [unwired: 1 in]
      n129 = Insert Into Array(array=w299, new element=w366) -> (w355:dbl[])  [unwired: 1 in]
      n130 = Insert Into Array(array=w300, new element=w367) -> (w354:dbl[])  [unwired: 1 in]
      n131 = Insert Into Array(array=w301, new element=w333) -> (w350:dbl[])  [unwired: 1 in]
      n132 = Insert Into Array(array=w302, new element=w328) -> (w314:dbl[])  [unwired: 1 in]
      n133 = Insert Into Array(array=w303, new element=w327) -> (w313:dbl[])  [unwired: 1 in]
      n134 = Insert Into Array(array=w304, new element=w326) -> (w312:dbl[])  [unwired: 1 in]
      n135 = Insert Into Array(array=w305, new element=w325) -> (w311:dbl[])  [unwired: 1 in]
    }
    n136 = Array Max & Min(array=w226) -> (min value=w233:dbl)  [unwired: 3 out]
    n137 = Array Max & Min(array=w225) -> (min value=w231:dbl)  [unwired: 3 out]
    n138 = Array Max & Min(array=w224) -> (min value=w229:dbl)  [unwired: 3 out]
    n139 = Array Max & Min(array=w223) -> (min value=w227:dbl)  [unwired: 3 out]
    n140 = Array Max & Min(array=w191) -> (min value=w213:dbl)  [unwired: 3 out]
    n141 = Array Max & Min(array=w192) -> (min value=w211:dbl)  [unwired: 3 out]
    n142 = Array Max & Min(array=w193) -> (min value=w209:dbl)  [unwired: 3 out]
    n143 = Array Max & Min(array=w194) -> (min value=w207:dbl)  [unwired: 3 out]
    n144 = Array Max & Min(array=w195) -> (min value=w239:dbl)  [unwired: 3 out]
    n145 = Array Max & Min(array=w196) -> (min value=w208:dbl)  [unwired: 3 out]
    n146 = Array Max & Min(array=w197) -> (min value=w210:dbl)  [unwired: 3 out]
    n147 = Array Max & Min(array=w198) -> (min value=w212:dbl)  [unwired: 3 out]
    n148 = Array Max & Min(array=w204) -> (min value=w214:dbl)  [unwired: 3 out]
    n149 = Array Max & Min(array=w219) -> (min value=w228:dbl)  [unwired: 3 out]
    n150 = Array Max & Min(array=w220) -> (min value=w230:dbl)  [unwired: 3 out]
    n151 = Array Max & Min(array=w221) -> (min value=w232:dbl)  [unwired: 3 out]
    n152 = Array Max & Min(array=w222) -> (min value=w234:dbl)  [unwired: 3 out]
    n153 = Less?(x=w239, y=3000.0) -> (x < y?=w238:bool)
    n154 = Select(t=w239, s=w238, f=inf) -> (s? t:f=w240:dbl)
    n155 = Build Array(w240, w207, w208, w209, w210, w211, w212, w213, w214, w227, w228, w229, w230, w231, w232, w233, w234) -> (w206:dbl[])
    n156 = Array Max & Min(array=w206) -> (max value=w235:dbl, max index (indices)=w215:i32)  [unwired: 2 out]
    n157 = case shown="1" w215 {
      tunnel: [90.0 95.0 85.0 100.0 80.0 120.0 60.0 130.0 50.0 140.0 40.0 150.0 30.0 160.0 20.0 170.0 10.0] -> w216
      frame 0, Default {
      }
      frame 1 {
      }
      frame 2 {
      }
      frame 3 {
      }
      frame 4 {
      }
      frame 5 {
      }
      frame 6 {
      }
      frame 7 {
      }
      frame 8 {
      }
      frame 9 {
      }
      frame 10 {
      }
      frame 11 {
      }
      frame 12 {
      }
      frame 13 {
      }
      frame 14 {
      }
      frame 15 {
      }
      frame 16 {
      }
    }
    n158 = Less?(x=w235, y="length") -> (x < y?=→"VEstop":bool)
    n159 = Negate(x=w216) -> (-x=w217:dbl)
    n160 = Add(x=90.0, y=w217) -> (x+y=→"Anthena_Steer":dbl)
    n161 = expression code="(x/180.0)*pi" "degrees to radians"(w216) -> (w205:dbl)
    n162 = Polar To Re/Im(2:w205, 3:7000.0 ("r")) -> (0:w200:dbl, 1:w199:dbl)
    n163 = Build Array(w199, w185) -> (w201:dbl[])
    n164 = Build Array(w200, w185) -> (w202:dbl[])
    n165 = Bundle(w201, w202) -> (→"TargetDerection":cluster{dbl[], dbl[]})  [unwired: 1 in]
    n166 = local read "stop"() -> (w180:bool)
    "session out" <- w170
  }
  n167 = while {
    tunnel: path "C:/Users/JungiHong/OneDrive/Hongik/HI-RACE/2026-01/platform_1_5/ExperimentModules/StanleyFFTest/main0.py" ("module in") -> [w399]
    tunnel: "main" ("module out") -> [w398]
    tunnel: [w396] -> w3
    tunnel: [w395] -> w2
    stop <- "stop" stop-if-true
    # "VisionSteering"
    n168 = Tick Count (ms)() -> (millisecond timer value=w433:u32)
    n169 = local read "session out"() -> (w397:refnum<k35>)
    n170 = feedback #3(u32 0 ("millisecond timer value")) -> (w432:u32)
    n171 = feedback-in #3(w433) -> ()
    n172 = Subtract(x=w433, y=w432) -> (x-y=→"CV Loop Time":u32)
    n173 = local read "Image_String"() -> (w400:string)
    n174 = Wait (ms)(milliseconds to wait=u32 30) -> ()  [unwired: 1 out]
    n175 = node(w397, w399, w398, string[] [] ("appended array"), w400) -> (w396:refnum<k35>, w395:errorcluster, w402:string[])  [unwired: 2 in, 2 out]
    "error out" <- w395
    n176 = Index Array(array=w402) -> (element #1=w420:string, element #2=w419:string, element #3=w421:string, element #4=w422:string, element #5=w423:string, element #6=w424:string, element #7=→"inference time":string)  [unwired: 8 in, 1 out]
    n177 = call "picturebox.vi"("s"=w422, "PictureBox"="Left_lane") -> ()  [unwired: 10 in]
    n178 = call "picturebox.vi"("s"=w423, "PictureBox"="Right_lane") -> ()  [unwired: 10 in]
    n179 = call "picturebox.vi"("s"=w424, "PictureBox"="Current_image") -> ()  [unwired: 10 in]
    n180 = Fract/Exp String To Number(string=w420) -> (number=w418:dbl)  [unwired: 3 in, 1 out]
    n181 = Fract/Exp String To Number(string=w419) -> (number=w412:dbl)  [unwired: 3 in, 1 out]
    n182 = Fract/Exp String To Number(string=w421) -> (number=w417:dbl)  [unwired: 3 in, 1 out]
    n183 = local read "Anthena_Steer"() -> (w405:i32)
    n184 = Less?(x=w412, y="ctelim") -> (x < y?=w409:bool)
    n185 = Not Equal?(x=w412, y=0.0) -> (x != y?=w410:bool)
    n186 = call "StanleyMethod.vi"("ψ(Heading Err)radian"=w418, "e(Cross-Track Err)m/s"=w412, "kappa"=w417, "v(Velocity)m/s"="v(Velocity)m/s", "k(Gain)"="k(Gain)") -> ("δ(OutputSteer)degrees"=w414:dbl)  [unwired: 1 out]
    n187 = And(x=w410, y=w409) -> (x .and. y?=w408:bool)
    n188 = local read "TooClose"() -> (w407:bool)
    n189 = local read "NearSteer"() -> (w406:dbl)
    n190 = Select(t=w414, s=w408, f=w405) -> (s? t:f=w404:dbl)
    n191 = Select(t=w406, s=w407, f=w404) -> (s? t:f=→"δ(OutputSteer)degrees":dbl)
  }
  n192 = while {
    tunnel: w56 -> [w448]
    tunnel: w36 -> [w447]
    tunnel: w33 -> [w446]
    tunnel: [w438] -> w31
    stop <- w453 stop-if-true
    w443 = T9 {"Global Rectangle"=[0, 50, 640, 360], "Contours"=[{"ID"=enum."External", "Type"=3, "Coordinates"=[0, 50, 640, 360]}]}  # ROI Descriptor
    n193 = case shown="False" "UseVideo" {
      tunnel: w448 -> [w456 w463]
      tunnel: [w458 w462] -> w436
      tunnel: [w457 w461] -> w441
      tunnel: w447 -> [_ w460]
      tunnel: w446 -> [w454 w459]
      frame False {
        n194 = call "IMAQ ReadFile 2"("File Path"="File Path", "error in (no error)"=w454, "Image"=w456) -> ("error out"=w458:errorcluster, "Image Out"=w457:T8)  [unwired: 4 in, 3 out]
      }
      frame True {
        n195 = call <vilib>:"IMAQdx Grab2.vi"("error in"=w459, "Image In"=w463, "Session In"=w460) -> ("error out"=w462:errorcluster, "Image Out"=w461:T8)  [unwired: 5 in, 2 out]
      }
    }
    n196 = Tick Count (ms)() -> (millisecond timer value=w449:u32)
    n197 = feedback #4(u32 0 ("millisecond timer value")) -> (w450:u32)
    n198 = feedback-in #4(w449) -> ()
    n199 = Subtract(x=w449, y=w450) -> (x-y=→"changearray":u32)
    n200 = call <vilib>:"IVA Mask from ROI.vi"("Shrink"=TRUE, "ROI Descriptor"=w443, "error in (no error)"=w436, "Out / In"=FALSE, "Image Src"=w441) -> ("error out"=w435:errorcluster, "Image Out"=w439:T8)  [unwired: 5 out]
    n201 = call-poly "IMAQ Write String"("error in (no error)"=w435, "Image Quality"=u32 500, "Image"=w439) -> ("error out"=w438:errorcluster, "FileString"=→"Image_String":string)  [unwired: 6 in, 1 out]
    n202 = local read "stop"() -> (w453:bool)
  }
  "error out 3" <- w31
  n203 = while {
    tunnel: w53 -> [w482]
    tunnel: w52 -> [w481]
    tunnel: [w475] -> w51
    tunnel: [w474] -> w50
    shift-right: [w469] -> _
    shift-left: w48 -> [w472]
    tunnel: w38 -> [w470]
    i -> [w476]
    stop <- w464 stop-if-true
    # "ERP_Racing Control"
    n204 = flat-sequence {
      tunnel: [w525] -> w479
      tunnel: [w524] -> w477
      tunnel: w482 -> [w527]
      tunnel: w481 -> [w526]
      tunnel: w476 -> [w523]
      tunnel: [w522] -> w473
      tunnel: w472 -> [w522]
      tunnel: w470 -> [w521]
      tunnel: [w531] -> w480
      tunnel: w479 -> [w531]
      tunnel: [w530] -> w478
      tunnel: w477 -> [w530]
      tunnel: w473 -> [w528]
      tunnel: [w528] -> w471
      tunnel: w480 -> [w559]
      tunnel: w478 -> [w558]
      tunnel: [w576] -> w475
      tunnel: [w575] -> w474
      tunnel: w471 -> [w550]
      tunnel: [w548] -> w469
      frame #0 {
        # "HENES RS232 프로토콜\nPC → 플랫폼"
        n205 = local read "δ(OutputSteer)degrees"() -> (w483:dbl)
        n206 = To Unsigned Byte Integer(number=w523) -> (unsigned 8bit integer=w510:u8)
        n207 = expression code="x*100"(w483) -> (w485:dbl)
        n208 = Boolean To (0,1)(Boolean="HLV_E-stop") -> (0, 1=w505:i16)
        n209 = Boolean To (0,1)(Boolean="HLV_A/M") -> (0, 1=w506:i16)
        n210 = To Word Integer(number=w485) -> (16bit integer=w488:i16)
        n211 = To Unsigned Byte Integer(number=w505) -> (unsigned 8bit integer=w503:u8)
        n212 = To Unsigned Byte Integer(number=w506) -> (unsigned 8bit integer=w504:u8)
        n213 = To Word Integer(number="input_spd") -> (16bit integer=w497:i16)
        n214 = In Range and Coerce(upper limit=i16 1999 ("상위 리미트"), x=w488, lower limit=i16 -1999 ("상위 리미트")) -> (coerced(x)=w496:i16)  [unwired: 1 out]
        n215 = Bundle By Name(cluster=w521, "HENES_M/A"=w504, "HENES_E-Stop"=w503, "HENES_Gear"="HLV_Gear", "HENES_Speed"=w497, "HENES_Steer"=w496, "HENES_Alive"=w510) -> (w514:T4)
        n216 = Unbundle By Name(w514) -> ("HENES_M/A"=w500:u8, "HENES_E-Stop"=w499:u8, "HENES_Gear"=w489:u8, "HENES_Speed"=w492:i16, "HENES_Steer"=w495:i16, "HENES_Alive"=w509:u8)
        n217 = Split Number(x=w495) -> (hi(x)=w494:u8, lo(x)=w493:u8)
        n218 = Split Number(x=w492) -> (hi(x)=w491:u8, lo(x)=w490:u8)
        n219 = Replace Array Subset(array=u8[] [83, 84, 88, 0, 0, 0, 0, 0, 0, 0, 0, 13, 10] ("unsigned byte array"), new element #1=w500, index #1=3, new element #2=w499, index #2=4, new element #3=w489, index #3=5, new element #4=w491, index #4=6, new element #5=w490, index #5=7, new element #6=w494, index #6=8, new element #7=w493, index #7=9, new element #8=w509, index #8=10) -> (w512:u8[])
        n220 = Byte Array To String(unsigned byte array=w512) -> (string=w511:string)
        n221 = VISA Write(VISA resource name=w527, write buffer=w511, error in (no error)=w526) -> (VISA resource name out=w525:refnum<visa-resource-name>, error out=w524:errorcluster)  [unwired: 1 out]
      }
      frame #1 {
        n222 = Wait Until Next ms Multiple(millisecond multiple=u32 20 ("대기 시간 (ms)")) -> ()  [unwired: 1 out]
      }
      frame #2 {
        # "HENES RS232 프로토콜\n플랫폼 → PC"
        n223 = property class="Instr"(reference=w559, error in=w558) -> (reference out=w539:refnum<visa-resource-name>, error out=w538:errorcluster, "Serial Settings:Number of Bytes at Serial Port"=w537:u32)
        n224 = Greater?(x=w537, y=u32 14) -> (0:w555:bool)
        n225 = case shown="True" w555 {
          tunnel: w539 -> [w603 w608]
          tunnel: w538 -> [w602 w607]
          tunnel: [w603 w606] -> w557
          tunnel: [w602 w605] -> w556
          tunnel: w537 -> [_ w604]
          frame False {
          }
          frame True {
            n226 = VISA Read(VISA resource name=w608, byte count=w604, error in (no error)=w607) -> (VISA resource name out=w606:refnum<visa-resource-name>, error out=w605:errorcluster)  [unwired: 2 out]
          }
        }
        n227 = VISA Read(VISA resource name=w557, byte count=u32 13, error in (no error)=w556) -> (VISA resource name out=w576:refnum<visa-resource-name>, read buffer=w574:string, error out=w575:errorcluster)  [unwired: 1 out]
        "버퍼 읽기" <- w574
        n228 = Match Pattern(string=w574, regular expression="STX") -> (match substring=w571:string, after substring=w572:string)  [unwired: 1 in, 2 out]
        n229 = Concatenate Strings(w571, w572) -> (w570:string)
        n230 = String To Byte Array(string=w570) -> (unsigned byte array=w552:u8[])
        n231 = Index Array(array=w552, index #1=0, index #2=1, index #3=2) -> (element #1=w565:u8, element #2=w564:u8, element #3=w563:u8)
        n232 = Build Array(w565, w564, w563) -> (w562:u8[])
        n233 = Byte Array To String(unsigned byte array=w562) -> (string=w560:string)
        n234 = Equal?(x="STX", y=w560) -> (x = y?=w551:bool)
        n235 = case shown="True" w551 {
          tunnel: w552 -> [_ w601]
          tunnel: [w578 w588] -> w548
          tunnel: w550 -> [w578 w590]
          frame False {
          }
          frame True {
            n236 = Index Array(array=w601, index #1=3, index #2=4, index #3=5, index #4=6, index #5=7, index #6=8, index #7=9, index #8=10) -> (element #1=w589:u8, element #2=w587:u8, element #3=w586:u8, element #4=w585:u8, element #5=w584:u8, element #6=w582:u8, element #7=w581:u8, element #8=w579:u8)
            n237 = Join Numbers(hi=w585, lo=w584) -> ((hi.lo)=w592:u16)
            n238 = Join Numbers(hi=w582, lo=w581) -> ((hi.lo)=w591:u16)
            n239 = To Word Integer(number=w592) -> (16bit integer=w583:i16)
            n240 = To Word Integer(number=w591) -> (16bit integer=w580:i16)
            n241 = Bundle By Name(cluster=w590, "HLV_M/A_Status"=w589, "HLV_E-Stop"=w587, "HLV_Gear"=w586, "HLV_Speed"=w583, "HLV_Steer"=w580, "HLV_Alive"=w579) -> (w588:T7)
          }
        }
        n242 = Unbundle By Name(w548) -> ("HLV_M/A_Status"=w549:u8, "HLV_E-Stop"=w543:u8, "HLV_Gear"=→"Gear_Feed":u8, "HLV_Speed"=w541:i16, "HLV_Steer"=w540:i16, "HLV_Alive"=→"Alive_PCU":u8)
        n243 = To Double Precision Float(number=w541) -> (double precision float=w553:dbl)
        n244 = To Double Precision Float(number=w540) -> (double precision float=w546:dbl)
        n245 = Not Equal To 0?(x=w549) -> (x != 0?=→"Remote_M/A":bool)
        n246 = Not Equal To 0?(x=w543) -> (x != 0?=→"E-STOP":bool)
        n247 = expression code="x*0.01"(w553) -> (w532:dbl)
        "Speed_Feed(RPM)" <- w532
        n248 = expression code="x*0.01"(w546) -> (→"Steer_Feed":dbl)
        n249 = Divide(x=w532, y=60.0) -> (x/y=w536:dbl)
        n250 = Multiply(x=w536, y=0.848205) -> (x*y=→"Speed_Feed(m/s)":dbl)
      }
    }
    n251 = Tick Count (ms)() -> (millisecond timer value=w466:u32)
    n252 = feedback #5(u32 0 ("millisecond timer value")) -> (w467:u32)
    n253 = feedback-in #5(w466) -> ()
    n254 = Subtract(x=w466, y=w467) -> (x-y=→"HENES Loop Time":u32)
    n255 = local read "stop"() -> (w464:bool)
  }
  n256 = VISA Close(VISA resource name=w29, error in (no error)=w28) -> (error out=w30:errorcluster)
  n257 = call <vilib>:"Clear Errors.vi"("error in (no error)"=w30) -> ()  [unwired: 5 in, 2 out]
  n258 = while {
    stop <- w610 stop-if-true
    w613 = -450.0 ("element")
    w615 = 100.0 ("element")
    w614 = 450.0 ("element")
    w636 = 1200.0 ("f")
    w630 = 1200.0 ("element")
    w633 = 0.0 ("element")
    w637 = -300.0 ("element")
    w634 = 800.0 ("element")
    w638 = 100.0 ("element")
    w635 = 450.0 ("element")
    w627 = 0.0 ("element")
    w631 = -300.0 ("element")
    w628 = -800.0 ("element")
    w632 = 100.0 ("element")
    w629 = -450.0 ("element")
    # "뒤로 빠꾸"
    # "가까운 실제 존재 장애물은 피하기"
    # "Neer Steering"
    n259 = local read "X_arraysREAL"() -> (w612:i32[])
    n260 = local read "Y_arraysREAL"() -> (w611:i32[])
    n261 = local read "GoBack"() -> (w609:bool)
    n262 = Select(t=1700.0, s=w609, f=950.0 ("element")) -> (s? t:f=w626:dbl)
    n263 = Build Array(w629, w629, w628, w628, w627, w627, w629) -> (w652:dbl[])
    n264 = Build Array(w632, w631, w631, w630, w630, w632, w632) -> (w651:dbl[])
    n265 = Build Array(w635, w635, w634, w634, w633, w633, w635) -> (w644:dbl[])
    n266 = Build Array(w638, w637, w637, w636, w636, w638, w638) -> (w645:dbl[])
    n267 = Build Array(w614, w614, w613, w613, w614) -> (w623:dbl[])
    n268 = Build Array(w615, w626, w626, w615, w615) -> (w622:dbl[])
    n269 = call "ROI_IN_Check.vi"("도형Y좌표"=w651, "도형X좌표"=w652, "LiDAR_Y"=w611, "LiDAR_X"=w612) -> ("ROI_IN_Y"=w654:i32[], "ROI_IN_X"=w653:i32[])  [unwired: 6 in]
    n270 = Bundle(w652, w651) -> (→"NearCarROILeft":cluster{dbl[], dbl[]})  [unwired: 1 in]
    n271 = call "ROI_IN_Check.vi"("도형Y좌표"=w645, "도형X좌표"=w644, "LiDAR_Y"=w611, "LiDAR_X"=w612) -> ("ROI_IN_Y"=w657:i32[], "ROI_IN_X"=w656:i32[])  [unwired: 6 in]
    n272 = Bundle(w644, w645) -> (→"NearCarROIRight":cluster{dbl[], dbl[]})  [unwired: 1 in]
    n273 = call "ROI_IN_Check.vi"("도형Y좌표"=w622, "도형X좌표"=w623, "LiDAR_Y"=w611, "LiDAR_X"=w612) -> ("ROI_IN_Y"=w619:i32[], "ROI_IN_X"=w620:i32[])  [unwired: 6 in]
    n274 = Bundle(w623, w622) -> (→"GobackROI":cluster{dbl[], dbl[]})  [unwired: 1 in]
    n275 = Bundle("ROI_IN_X"=w653, "ROI_IN_Y"=w654) -> (→"NearCarPointsLeft":cluster{"ROI_IN_X":i32[], "ROI_IN_Y":i32[]})  [unwired: 1 in]
    n276 = Bundle("ROI_IN_X"=w656, "ROI_IN_Y"=w657) -> (→"NearCarPointsRight":cluster{"ROI_IN_X":i32[], "ROI_IN_Y":i32[]})  [unwired: 1 in]
    n277 = Re/Im To Polar(2:w654, 3:w653) -> (1:w655:dbl[])  [unwired: 1 out]
    n278 = Re/Im To Polar(2:w657, 3:w656) -> (1:w658:dbl[])  [unwired: 1 out]
    n279 = Re/Im To Polar(2:w619, 3:w620) -> (1:w618:dbl[])  [unwired: 1 out]
    n280 = Array Max & Min(array=w655) -> (min value=w659:dbl)  [unwired: 3 out]
    n281 = Array Size(array=w655) -> (size(s)=w650:i32)
    n282 = Array Max & Min(array=w658) -> (min value=w660:dbl)  [unwired: 3 out]
    n283 = Array Size(array=w658) -> (size(s)=w643:i32)
    n284 = Array Size(array=w618) -> (size(s)=w624:i32)
    n285 = Divide(x=40000.0, y=w659) -> (x/y=w662:dbl)
    n286 = Not Equal To 0?(x=w650) -> (x != 0?=w667:bool)
    n287 = Divide(x=-40000.0, y=w660) -> (x/y=w664:dbl)
    n288 = Not Equal To 0?(x=w643) -> (x != 0?=w666:bool)
    n289 = Not Equal To 0?(x=w624) -> (x != 0?=w625:bool)
    n290 = Select(t=w662, s=w667, f=0.0) -> (s? t:f=w663:dbl)
    n291 = Select(t=w664, s=w666, f=0.0) -> (s? t:f=w665:dbl)
    n292 = Or(x=w667, y=w666) -> (x .or. y?=→"TooClose":bool)
    n293 = Add(x=w663, y=w665) -> (x+y=→"NearSteer":dbl)
    n294 = local write "GoBack"(w625) -> ()
    n295 = local read "stop"() -> (w610:bool)
  }
  n296 = Close Python Session(session in=w3, error in=w2) -> (11:→"error out 2":errorcluster)
  n297 = Close Python Session(session in=w14, error in=w15) -> (11:→"Clustering Error":errorcluster)
  n298 = VISA Flush I/O Buffer(VISA resource name=w51, error in (no error)=w50) -> (VISA resource name out=w54:refnum<visa-resource-name>, error out=w55:errorcluster)  [unwired: 1 in]
  n299 = VISA Close(VISA resource name=w54, error in (no error)=w55) -> (error out=w49:errorcluster)
  n300 = call <vilib>:"Simple Error Handler.vi"("error in (no error)"=w49) -> ()  [unwired: 4 in, 5 out]
